vi "CRYScale Style Menu.vi"(11 "ScaleStyle In":u8) -> (3 "ScaleStyle Out":u8)   [LabVIEW 2013]
panel:
  out "Interpolation":string
  in  "ScaleStyle8":bool
  in  "ScaleStyle7":bool
  in  "ScaleStyle6":bool
  in  "ScaleStyle5":bool
  in  "ScaleStyle4":bool
  in  "ScaleStyle3":bool
  in  "ScaleStyle2":bool
  in  "ScaleStyle1":bool
  in  "ScaleStyle0":bool
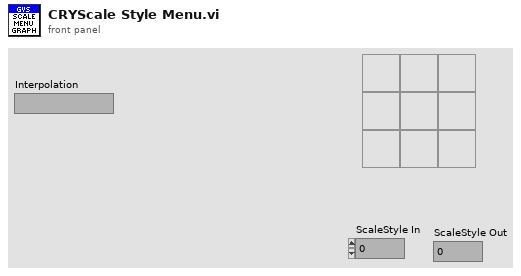
[diagram p1: front panel]
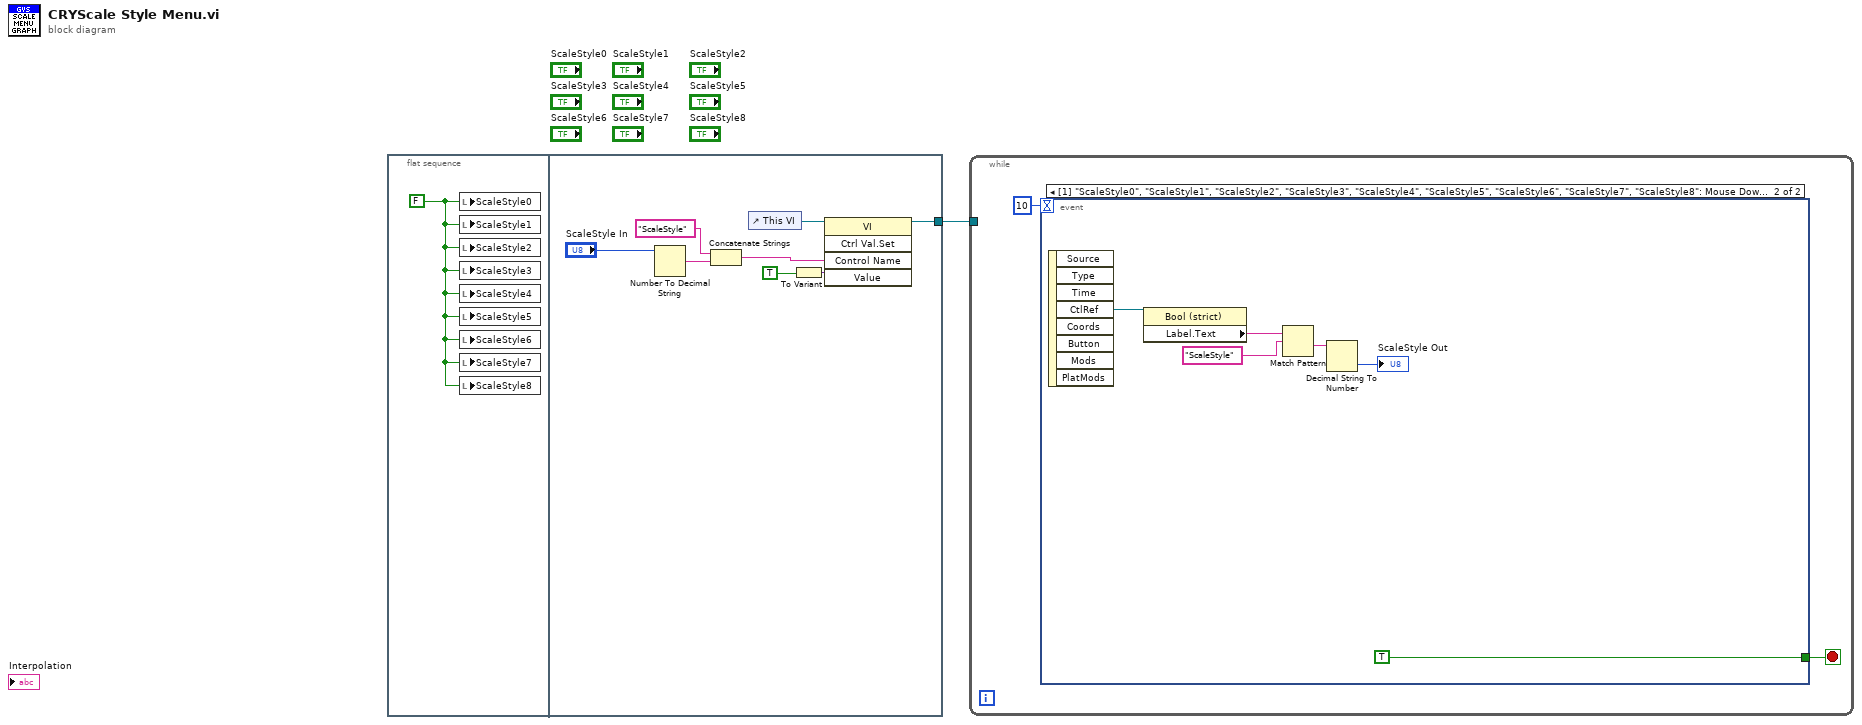
[diagram p0: block diagram]
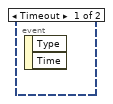
[diagram p2: hidden frame]
diagram:
  n1 = flat-sequence {
    tunnel: [w3] -> w1
    frame #0 {
      w2 = FALSE ("ScaleStyle0")
      n2 = local write "ScaleStyle0"(w2) -> ()
      n3 = local write "ScaleStyle1"(w2) -> ()
      n4 = local write "ScaleStyle2"(w2) -> ()
      n5 = local write "ScaleStyle3"(w2) -> ()
      n6 = local write "ScaleStyle4"(w2) -> ()
      n7 = local write "ScaleStyle5"(w2) -> ()
      n8 = local write "ScaleStyle6"(w2) -> ()
      n9 = local write "ScaleStyle7"(w2) -> ()
      n10 = local write "ScaleStyle8"(w2) -> ()
    }
    frame #1 {
      n11 = Number To Decimal String(number="ScaleStyle In") -> (decimal integer string=w8:string)  [unwired: 1 out]
      n12 = Concatenate Strings("ScaleStyle", w8) -> (w5:string)
      n13 = control-ref of="This VI"() -> (w4:refnum<vi>)
      n14 = To Variant(anything=TRUE) -> (Variant=w6:variant)
      n15 = invoke class="VI" method="Ctrl Val.Set"(reference=w4, "Control Name"=w5, "Value"=w6) -> (reference out=w3:refnum<vi>)  [unwired: 2 in, 4 out]
    }
  }
  n16 = while {
    tunnel: w1 -> [_]
    stop <- w11 stop-if-true
    n17 = event shown="[1] \"ScaleStyle0\", \"ScaleStyle1\", \"ScaleStyle2\", \"ScaleStyle3\", \"ScaleStyle4\", \"ScaleStyle5\", \"ScaleStyle6\", \"ScaleStyle7\", \"ScaleStyle8\": Mouse Down" {
      selector: _ -> [_ _]
      dyn-events: _ -> [_ _]
      timeout: 10 -> [_ _]
      tunnel: [_ TRUE] -> w11
      event Timeout {
        n18 = event-data() -> ()  [unwired: 3 out]
      }
      event "ScaleStyle0", "ScaleStyle1", "ScaleStyle2", "ScaleStyle3", "ScaleStyle4", "ScaleStyle5", "ScaleStyle6", "ScaleStyle7", "ScaleStyle8": Mouse Down {
        n19 = event-data() -> ("CtlRef"=w18:refnum<vi>)  [unwired: 8 out]
        n20 = property class="Bool (strict)"(reference=w18) -> ("Label.Text"=w15:string)  [unwired: 1 in, 2 out]
        n21 = Match Pattern(string=w15, regular expression="ScaleStyle") -> (after substring=w16:string)  [unwired: 4 out]
        n22 = Decimal String To Number(string=w16) -> (number=→"ScaleStyle Out":i32)  [unwired: 3 out]
      }
    }
  }
